vi "Set Voltage.vi"(8 "error in (no error)":errorcluster, 10 "Voltage":dbl, 11 "PS Test in":refnum<class "PS Test.lvclass">) -> (0 "error out":errorcluster, 3 "PS Test out":refnum<class "PS Test.lvclass">)   [LabVIEW 2021, in "PS.lvlib" / "PS Test.lvclass"]
uses:
  PS Test.lvclass
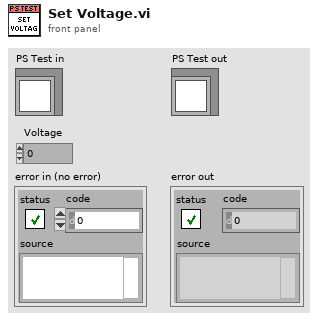
[diagram p1: front panel]
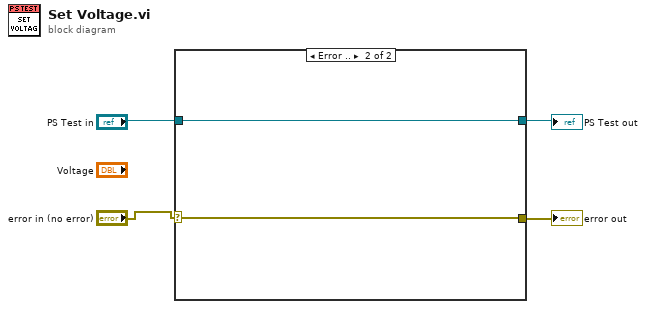
[diagram p0: block diagram]
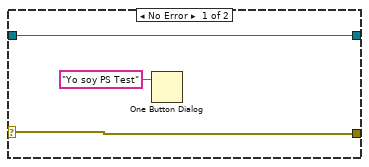
[diagram p2: hidden frame]
diagram:
  n1 = case shown="Error .." "error in (no error)" {
    selector: "error in (no error)" -> [w6 w8]
    tunnel: [w7 w9] -> w4
    tunnel: "PS Test in" -> [w7 w9]
    tunnel: [w6 w8] -> w1
    frame No Error {
      n2 = One Button Dialog(message="Yo soy PS Test") -> ()  [unwired: 1 in, 1 out]
    }
    frame Error {
    }
  }
  "error out" <- w1
  "PS Test out" <- w4
